vi "Voltage Nominal Write Array.vi"(8 "error in":errorcluster, 10 "Voltage Nominal AV":dbl[](array[numeric]), 11 "Cycler in":refnum<class "Cycler.lvclass">) -> (0 "error out":errorcluster, 3 "Cycler out":refnum<class "Cycler.lvclass">)   [LabVIEW 2023, in "Cycler.lvclass"]
uses:
  Cycler.lvclass
  Cycler.lvclass/Cycler.ctl
  Low Level Capabilities/Voltage/Voltage Nominal Value/Voltage Nominal Value.lvclass
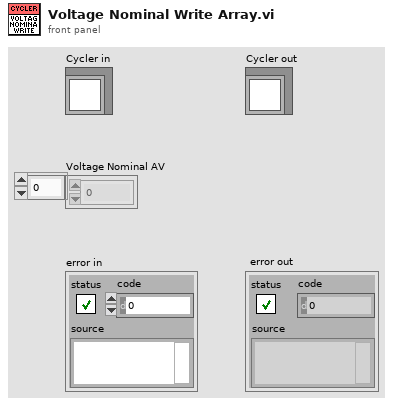
[diagram p1: front panel]
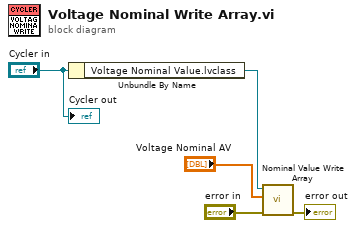
[diagram p0: block diagram]
diagram:
  n1 = Unbundle By Name("Cycler in") -> ("Voltage Nominal Value.lvclass"=w1:refnum<class "Voltage Nominal Value.lvclass">)
  n2 = call-dynamic "Nominal Value Write Array.vi"("Voltage Nominal Value in"=w1, "Voltage Nominal Value Value"="Voltage Nominal AV", "error in"="error in") -> ("error out"=→"error out":errorcluster)  [unwired: 6 in, 1 out]
  "Cycler out" <- "Cycler in"
